vi "FFT.vi"() -> ()   [LabVIEW 2020]
uses:
  <vilib>/Analysis/NI_AALPro.lvlib
panel:
  out "Waveform Graph":dbl[](graph)
  in  "Number of sample":i32
  in  "Frequency":i32
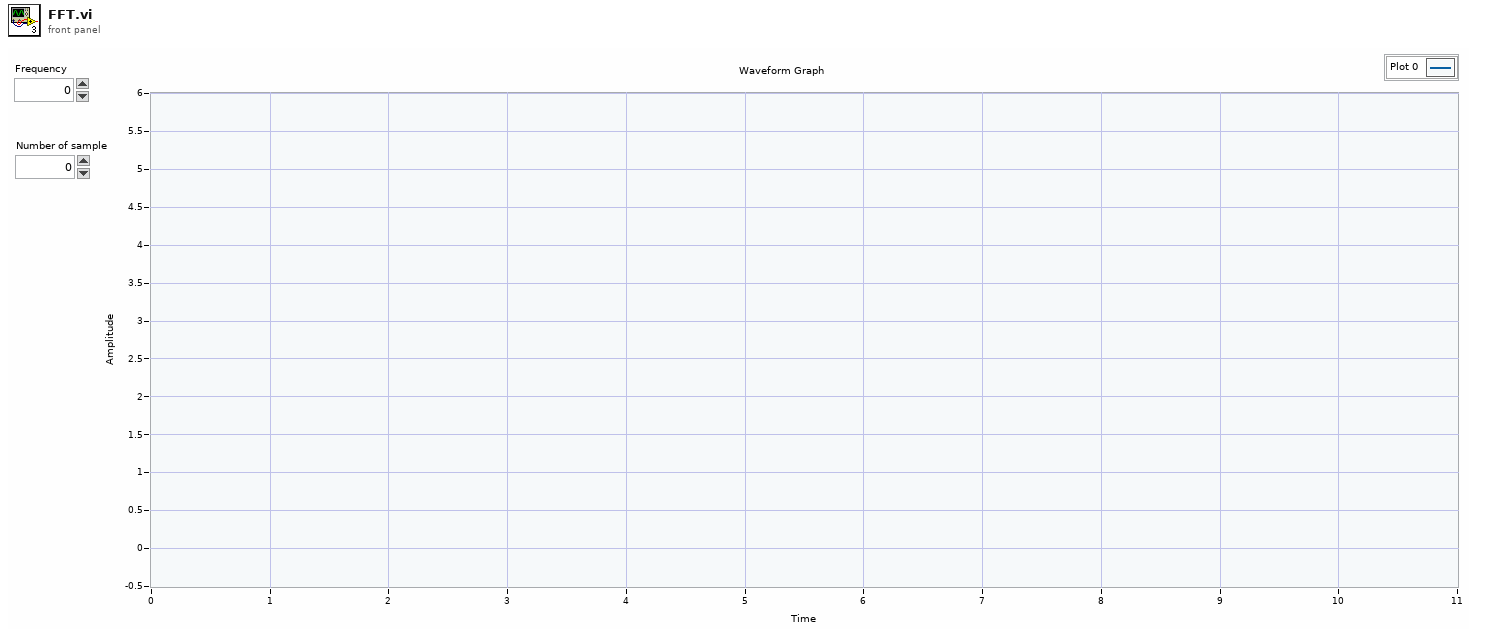
[diagram p1: front panel]
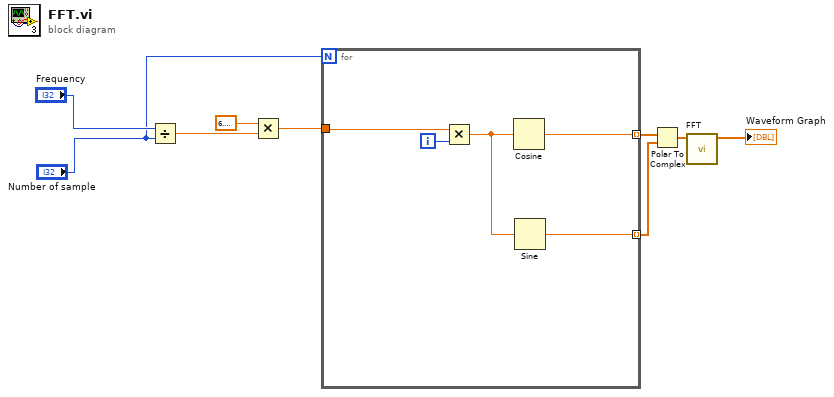
[diagram p0: block diagram]
diagram:
  n1 = Divide(x="Frequency", y="Number of sample") -> (x/y=w3:dbl)
  n2 = Multiply(x=6.283185307179586, y=w3) -> (x*y=w7:dbl)
  n3 = for {
    N: "Number of sample" -> [_]
    tunnel: w7 -> [w14]
    tunnel: [w12] -> w6 mode=indexing
    tunnel: [w11] -> w5 mode=indexing
    i -> [w13]
    n4 = Multiply(x=w14, y=w13) -> (x*y=w10:dbl)
    n5 = Cosine(x=w10) -> (cos(x)=w12:dbl)
    n6 = Sine(x=w10) -> (sin(x)=w11:dbl)
  }
  n7 = Polar To Complex(1:w5, 2:w6) -> (0:w4:cdb[])
  n8 = call-poly <vilib>:"FFT.vi"("X"=w4) -> ("FFT {X}"=→"Waveform Graph":cdb[])  [unwired: 9 in, 1 out]
